vi "Align Rectangles.vi"(6 "Offset":cluster{"X":dbl, "Y":dbl}, 8 "Position 2 [Top-Left]":T3, 9 "rect 2":T2, 10 "Position 1 [Top-Left]":T3, 11 "rect 1":T2) -> (1 "rect out":T2)   [LabVIEW 2023]
doc: "Given bounds of two rectangles. calculates positoin of rect 2 to be aligned with rectangle one as specified. (Rect2 bounds will be converted to dimensions, so if you only have the rectabgle width and height, you cna provide just the right and bottom coords.)\n\nAn optional padding can applied to offset the second rectangle from the first."
uses:
  controls/corner position.ctl
  Controls/x,y cluster_DBL.ctl
panel:
  out "select position of first rect":T1 {"Y" format="%.3f"; "X" format="%.3f"}
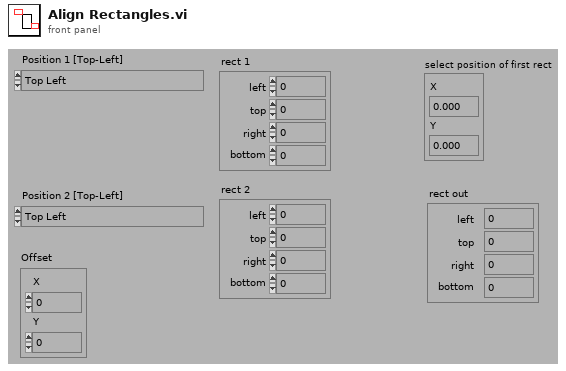
[diagram p1: front panel]
types:
  T1 = typedef "x,y cluster_DBL.ctl" = cluster{"X":dbl, "Y":dbl}
  T2 = cluster{"left":i16, "top":i16, "right":i16, "bottom":i16}
  T3 = typedef "corner position.ctl" = enum16{"Top Left", "Bottom Left", "Top Right", "Bottom Right", "Center"}
  T4 = typedef "Rect or Line Cluster.ctl" = cluster{"left":dbl, "top":dbl, "right":dbl, "bottom":dbl}
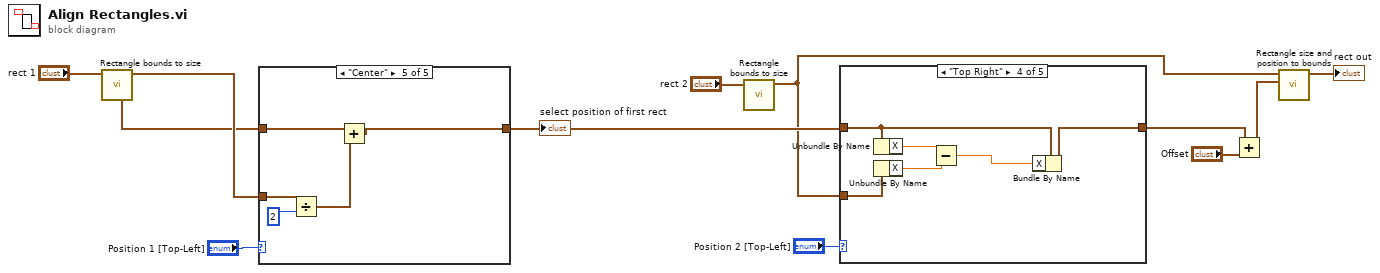
[diagram p0: block diagram]
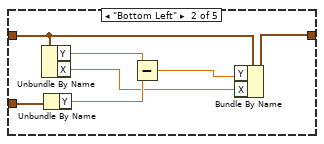
[diagram p3: hidden frame]
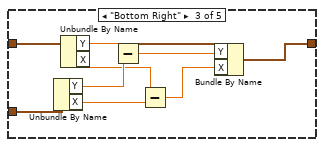
[diagram p4: hidden frame]
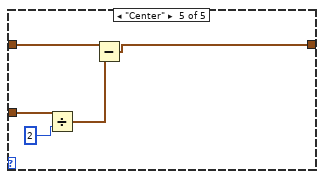
[diagram p5: hidden frame]
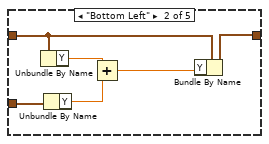
[diagram p7: hidden frame]
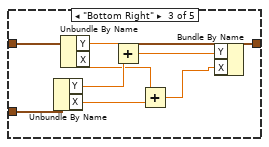
[diagram p8: hidden frame]
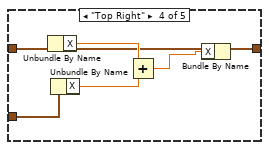
[diagram p9: hidden frame]
diagram:
  n1 = call "Rectangle bounds to size.vi"("bounds"="rect 1") -> ("size"=w8:T1, "left top"=w7:T1)  [unwired: 6 in, 3 out]
  n2 = case shown="\"Center\"" "Position 1 [Top-Left]" {
    tunnel: w7 -> [w13 w16 w21 w30 w37]
    tunnel: [w13 w14 w20 w29 w35] -> w11
    tunnel: w8 -> [_ w18 w25 w32 w39]
    frame "Top Left", Default {
    }
    frame "Bottom Left" {
      n3 = Unbundle By Name(w16) -> ("Y"=w19:dbl)
      n4 = Unbundle By Name(w18) -> ("Y"=w17:dbl)
      n5 = Add(x=w19, y=w17) -> (x+y=w15:dbl)
      n6 = Bundle By Name(cluster=w16, "Y"=w15) -> (w14:T1)
    }
    frame "Bottom Right" {
      n7 = Unbundle By Name(w25) -> ("Y"=w27:dbl, "X"=w23:dbl)
      n8 = Unbundle By Name(w21) -> ("Y"=w28:dbl, "X"=w24:dbl)
      n9 = Add(x=w28, y=w27) -> (x+y=w26:dbl)
      n10 = Add(x=w24, y=w23) -> (x+y=w22:dbl)
      n11 = Bundle By Name(cluster=w21, "Y"=w26, "X"=w22) -> (w20:T1)
    }
    frame "Top Right" {
      n12 = Unbundle By Name(w30) -> ("X"=w34:dbl)
      n13 = Unbundle By Name(w32) -> ("X"=w31:dbl)
      n14 = Add(x=w34, y=w31) -> (x+y=w33:dbl)
      n15 = Bundle By Name(cluster=w30, "X"=w33) -> (w29:T1)
    }
    frame "Center" {
      n16 = Divide(x=w39, y=2) -> (x/y=w36:T1)
      n17 = Add(x=w37, y=w36) -> (x+y=w35:T1)
    }
  }
  "select position of first rect" <- w11
  n18 = call "Rectangle bounds to size.vi"("bounds"="rect 2") -> ("size"=w4:T1)  [unwired: 6 in, 4 out]
  n19 = case shown="\"Top Right\"" "Position 2 [Top-Left]" {
    tunnel: w11 -> [w40 w44 w49 w58 w65]
    tunnel: [w40 w43 w48 w59 w63] -> w1
    tunnel: w4 -> [_ w46 w53 w61 w67]
    frame "Top Left", Default {
    }
    frame "Bottom Left" {
      n20 = Unbundle By Name(w44) -> ("Y"=w47:dbl, "X"=w41:dbl)
      n21 = Unbundle By Name(w46) -> ("Y"=w45:dbl)
      n22 = Subtract(x=w47, y=w45) -> (x-y=w42:dbl)
      n23 = Bundle By Name(cluster=w44, "Y"=w42, "X"=w41) -> (w43:T1)
    }
    frame "Bottom Right" {
      n24 = Unbundle By Name(w53) -> ("Y"=w55:dbl, "X"=w51:dbl)
      n25 = Unbundle By Name(w49) -> ("Y"=w56:dbl, "X"=w52:dbl)
      n26 = Subtract(x=w56, y=w55) -> (x-y=w54:dbl)
      n27 = Subtract(x=w52, y=w51) -> (x-y=w50:dbl)
      n28 = Bundle By Name(cluster=w49, "Y"=w54, "X"=w50) -> (w48:T1)
    }
    frame "Top Right" {
      n29 = Unbundle By Name(w58) -> ("X"=w62:dbl)
      n30 = Unbundle By Name(w61) -> ("X"=w60:dbl)
      n31 = Subtract(x=w62, y=w60) -> (x-y=w57:dbl)
      n32 = Bundle By Name(cluster=w58, "X"=w57) -> (w59:T1)
    }
    frame "Center" {
      n33 = Divide(x=w67, y=2) -> (x/y=w64:T1)
      n34 = Subtract(x=w65, y=w64) -> (x-y=w63:T1)
    }
  }
  n35 = Add(x=w1, y="Offset") -> (x+y=w2:T1)
  n36 = call "Rectangle size and position to bounds.vi"("Position"=w2, "Size"=w4) -> ("bounds"=→"rect out":T4)  [unwired: 8 in, 1 out]
